vi "openbci_parse_acc_data.vi"(11 "string_acc_data":string) -> (3 "acc_data":dbl[](array[numeric]))   [LabVIEW 2013]
doc: "For the Acceleration data values, data is transfered as a 16-bit integer"
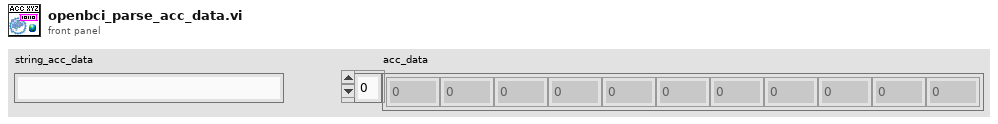
[diagram p1: front panel]
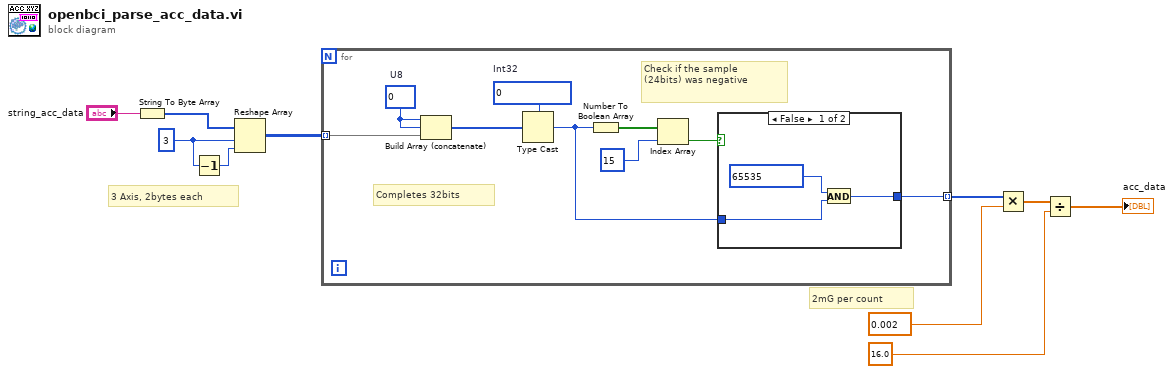
[diagram p0: block diagram]
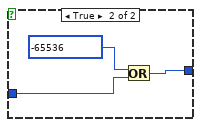
[diagram p2: hidden frame]
diagram:
  w7 = 3 ("dimension size")
  # "2mG per count"
  # "3 Axis, 2bytes each"
  n1 = String To Byte Array(string="string_acc_data") -> (unsigned byte array=w9:u8[])
  n2 = Decrement(x=w7) -> (x-1=w6:i32)
  n3 = Reshape Array(w9, w7, w6) -> (w8:u8[][])
  n4 = for {
    tunnel: w8 -> [w13] mode=indexing
    tunnel: [w11] -> w5 mode=indexing
    w19 = 0  # Int32
    w12 = u8 0  # U8
    # "Check if the sample\n(24bits) was negative"
    # "Completes 32bits"
    n5 = Build Array (concatenate)(w12, w12, w13) -> (w14:u8[])
    n6 = Type Cast(type=w19, x=w14) -> (*(type *) &x=w18:i32)
    n7 = Number To Boolean Array(number=w18) -> (Boolean array=w17:bool[])
    n8 = Index Array(array=w17, index=15) -> (element=w16:bool)
    n9 = case shown="False" w16 {
      tunnel: w18 -> [w21 w24]
      tunnel: [w20 w23] -> w11
      frame False {
        n10 = And(x=65535 ("dimension size"), y=w21) -> (x .and. y?=w20:i32)
      }
      frame True {
        n11 = Or(x=-65536 ("dimension size"), y=w24) -> (x .or. y?=w23:i32)
      }
    }
  }
  n12 = Multiply(x=w5, y=0.002) -> (x*y=w3:dbl[])
  n13 = Divide(x=w3, y=16.0) -> (x/y=→"acc_data":dbl[])
